vi "S4GUI_001.vi"() -> ()   [LabVIEW 2018] (continued)
            n2909 = call "Write WPROT.vi"("error in (no error)"=w7024, "Opt_Selector.lvclass"=w7023, "Instrument in"=w7042) -> ("error out"=w7021:errorcluster, "Instrument out"=w7022:refnum<class "Instrument.lvclass">)  [unwired: 7 in]
            n2910 = call "Write Instrument.lvclass.vi"("error in (no error)"=w7021, "Instrument.lvclass"=w7022, "S4ACS_GUI in"=w7040) -> ("error out"=w7043:errorcluster, "S4ACS_GUI out"=w7044:refnum<class "S4GUI.lvclass">)  [unwired: 7 in]
            n2911 = call-dynamic "Write ciclos.vi"("error in (no error)"=w7043, "ciclos"=u32 0, "S4ACS_GUI in"=w7044) -> ("error out"=w7017:errorcluster, "S4ACS_GUI out"=w7018:refnum<class "S4GUI.lvclass">)  [unwired: 7 in]
          }
          frame Enabled {
            w7133 = FALSE ("Wait Until Done")
            n2912 = call <vilib>:"Application Directory.vi"() -> ("Application Directory"=w7136:path)
            n2913 = Build Path(base path=w7136, name or relative path="MsgAbortSync.vi") -> (appended path=w7137:path)
            n2914 = Open VI Reference(vi path=w7137, error in (no error)=w7131) -> (vi reference=w7135:refnum<vi>, error out=w7134:errorcluster)  [unwired: 4 in]
            n2915 = invoke class="VI" method="Run VI"(reference=w7135, error in=w7134, "Wait until done"=w7133, "Auto Dispose Ref"=w7133) -> (error out=w7130:errorcluster)  [unwired: 1 in, 4 out]
          }
        }
        n2916 = property on="#Cycles Done" class="Slide (strict)"(error in=w7011, "Scale.Maximum"=w7013, "Scale.Minimum"=w7013) -> (error out=w7014:errorcluster)  [unwired: 1 in, 1 out]
      }
      event "Pause SM": Value Change {
        n2917 = event-data() -> ()  [unwired: 1 in, 6 out]
        n2918 = disable-structure shown="Enabled" {
          disable-tunnel: w7141 -> [w7153 w7162]
          disable-tunnel: w7140 -> [w7152 w7163]
          disable-tunnel: [w7143 w7162] -> w7139
          disable-tunnel: [w7142 w7161] -> w7138
          frame Disabled {
            n2919 = disable-structure shown="Enabled" {
              disable-tunnel: w7153 -> [w7157 w7160]
              disable-tunnel: w7152 -> [w7156 w7159]
              disable-tunnel: [w7155 w7160] -> w7146
              disable-tunnel: [w7154 w7159] -> w7145
              frame Disabled {
                n2920 = call-dynamic "Write paused.vi"("error in (no error)"=w7156, "paused"=TRUE ("stopped"), "S4ACS_GUI in"=w7157) -> ("error out"=w7154:errorcluster, "S4ACS_GUI out"=w7155:refnum<class "S4GUI.lvclass">)  [unwired: 7 in]
              }
              frame Enabled {
              }
            }
            n2921 = call-dynamic "Read Obs_state.vi"("error in (no error)"=w7145, "S4ACS_GUI in"=w7146) -> ("error out"=w7149:errorcluster, "Obs_state"=w7151:u32, "S4ACS_GUI out"=w7150:refnum<class "S4GUI.lvclass">)  [unwired: 7 in]
            n2922 = call-dynamic "Write Obs_prevstate.vi"("error in (no error)"=w7149, "Obs_prevstate"=w7151, "S4ACS_GUI in"=w7150) -> ("error out"=w7147:errorcluster, "S4ACS_GUI out"=w7148:refnum<class "S4GUI.lvclass">)  [unwired: 7 in]
            n2923 = call-dynamic "Write Obs_state.vi"("error in (no error)"=w7147, "Obs_state"=u32 400, "S4ACS_GUI in"=w7148) -> ("error out"=w7142:errorcluster, "S4ACS_GUI out"=w7143:refnum<class "S4GUI.lvclass">)  [unwired: 7 in]
          }
          frame Enabled {
            w7165 = FALSE ("Wait Until Done")
            n2924 = call <vilib>:"Application Directory.vi"() -> ("Application Directory"=w7168:path)
            n2925 = Build Path(base path=w7168, name or relative path="MsgPauseSync.vi") -> (appended path=w7169:path)
            n2926 = Open VI Reference(vi path=w7169, error in (no error)=w7163) -> (vi reference=w7167:refnum<vi>, error out=w7166:errorcluster)  [unwired: 4 in]
            n2927 = invoke class="VI" method="Run VI"(reference=w7167, error in=w7166, "Wait until done"=w7165, "Auto Dispose Ref"=w7165) -> (error out=w7161:errorcluster)  [unwired: 1 in, 4 out]
          }
        }
      }
      event "Abort ch1": Value Change {
        n2928 = event-data() -> ()  [unwired: 1 in, 6 out]
        n2929 = disable-structure shown="Enabled" {
          disable-tunnel: w7173 -> [w7206 w7228]
          disable-tunnel: w7172 -> [w7204 w7221]
          disable-tunnel: [w7186 w7220] -> w7171
          disable-tunnel: [w7174 w7228] -> w7170
          frame Disabled {
            # "Para movimento \nda lamina retardadora"
            # "Restaura a última sequência de lâminas"
            n2930 = call-dynamic "Read AcquisitionA.vi"("error in (no error)"=w7204, "S4ACS_GUI in"=w7206) -> ("error out"=w7209:errorcluster, "Acquisition.lvclass"=w7208:refnum<class "Acquisition.lvclass">, "S4ACS_GUI out"=w7205:refnum<class "S4GUI.lvclass">)  [unwired: 7 in]
            n2931 = call-dynamic "Read Channel.vi"("error in (no error)"=w7209, "Acquisition in"=w7208) -> ("error out"=w7211:errorcluster, "Channel.lvclass"=w7210:refnum<class "Channel.lvclass">, "Acquisition out"=w7217:refnum<class "Acquisition.lvclass">)  [unwired: 7 in]
            n2932 = call-dynamic "Read State Machine.vi"("error in (no error)"=w7211, "Device in"=w7210) -> ("error out"=w7213:errorcluster, "State Machine.lvclass"=w7212:refnum<class "State Machine.lvclass">, "Device out"=w7215:refnum<class "Channel.lvclass">)  [unwired: 7 in]
            n2933 = call "Next State.vi"("error in (no error)"=w7213, "New_State"=u32 80, "State Machine in"=w7212) -> ("error out"=w7216:errorcluster, "State Machine out"=w7214:refnum<class "State Machine.lvclass">)  [unwired: 7 in]
            n2934 = call-dynamic "Write State Machine.vi"("error in (no error)"=w7216, "State Machine.lvclass"=w7214, "Device in"=w7215) -> ("error out"=w7218:errorcluster, "Device out"=w7219:refnum<class "Channel.lvclass">)  [unwired: 7 in]
            n2935 = call-dynamic "Write Channel.vi"("error in (no error)"=w7218, "Channel.lvclass"=w7219, "Acquisition in"=w7217) -> ("error out"=w7201:errorcluster, "Acquisition out"=w7202:refnum<class "Acquisition.lvclass">)  [unwired: 7 in]
            n2936 = call-dynamic "Write Acq_state.vi"("error in (no error)"=w7201, "Acq_state"=u32 0, "Acquisition in"=w7202) -> ("error out"=w7200:errorcluster, "Acquisition out"=w7199:refnum<class "Acquisition.lvclass">)  [unwired: 7 in]
            n2937 = call-dynamic "Write AcquisitionA.vi"("error in (no error)"=w7200, "Acquisition.lvclass"=w7199, "S4ACS_GUI in"=w7205) -> ("error out"=w7187:errorcluster, "S4ACS_GUI out"=w7185:refnum<class "S4GUI.lvclass">)  [unwired: 7 in]
            n2938 = call "Read Instrument.lvclass.vi"("error in (no error)"=w7187, "S4ACS_GUI in"=w7185) -> ("error out"=w7194:errorcluster, "Instrument.lvclass"=w7197:refnum<class "Instrument.lvclass">, "S4ACS_GUI out"=w7198:refnum<class "S4GUI.lvclass">)  [unwired: 7 in]
            n2939 = call "Read WPROT.vi"("error in (no error)"=w7194, "Instrument in"=w7197) -> ("error out"=w7193:errorcluster, "Opt_Selector.lvclass"=w7195:refnum<class "Opt_Selector.lvclass">, "Instrument out"=w7196:refnum<class "Instrument.lvclass">)  [unwired: 7 in]
            n2940 = call-dynamic "Read sequencia_ant.vi"("error in (no error)"=w7193, "Opt_Selector in"=w7195) -> ("error out"=w7189:errorcluster, "sequencia_ant"=w7188:u16, "Opt_Selector out"=w7190:refnum<class "Opt_Selector.lvclass">)  [unwired: 7 in]
            n2941 = call-dynamic "Write sequencia.vi"("error in (no error)"=w7189, "sequencia"=w7188, "Opt_Selector in"=w7190) -> ("error out"=w7178:errorcluster, "Opt_Selector out"=w7179:refnum<class "Opt_Selector.lvclass">)  [unwired: 7 in]
            n2942 = call-dynamic "Read State Machine.vi"("error in (no error)"=w7178, "Device in"=w7179) -> ("error out"=w7181:errorcluster, "State Machine.lvclass"=w7184:refnum<class "State Machine.lvclass">, "Device out"=w7177:refnum<class "Opt_Selector.lvclass">)  [unwired: 7 in]
            n2943 = call "Next State.vi"("error in (no error)"=w7181, "New_State"=10, "State Machine in"=w7184) -> ("error out"=w7180:errorcluster, "State Machine out"=w7183:refnum<class "State Machine.lvclass">)  [unwired: 7 in]
            n2944 = call-dynamic "Write State Machine.vi"("error in (no error)"=w7180, "State Machine.lvclass"=w7183, "Device in"=w7177) -> ("error out"=w7175:errorcluster, "Device out"=w7176:refnum<class "Opt_Selector.lvclass">)  [unwired: 7 in]
            n2945 = call "Write WPROT.vi"("error in (no error)"=w7175, "Opt_Selector.lvclass"=w7176, "Instrument in"=w7196) -> ("error out"=w7192:errorcluster, "Instrument out"=w7191:refnum<class "Instrument.lvclass">)  [unwired: 7 in]
            n2946 = call "Write Instrument.lvclass.vi"("error in (no error)"=w7192, "Instrument.lvclass"=w7191, "S4ACS_GUI in"=w7198) -> ("error out"=w7186:errorcluster, "S4ACS_GUI out"=w7174:refnum<class "S4GUI.lvclass">)  [unwired: 7 in]
          }
          frame Enabled {
            w7223 = FALSE ("Wait Until Done")
            n2947 = call <vilib>:"Application Directory.vi"() -> ("Application Directory"=w7226:path)
            n2948 = Build Path(base path=w7226, name or relative path="MsgAbort1.vi") -> (appended path=w7227:path)
            n2949 = Open VI Reference(vi path=w7227, error in (no error)=w7221) -> (vi reference=w7225:refnum<vi>, error out=w7224:errorcluster)  [unwired: 4 in]
            n2950 = invoke class="VI" method="Run VI"(reference=w7225, error in=w7224, "Wait until done"=w7223, "Auto Dispose Ref"=w7223) -> (error out=w7220:errorcluster)  [unwired: 1 in, 4 out]
          }
        }
      }
      event "Abort ch2": Value Change {
        n2951 = event-data() -> ()  [unwired: 1 in, 6 out]
        n2952 = disable-structure shown="Enabled" {
          disable-tunnel: w7232 -> [w7265 w7280]
          disable-tunnel: w7231 -> [w7263 w7281]
          disable-tunnel: [w7245 w7279] -> w7230
          disable-tunnel: [w7233 w7280] -> w7229
          frame Disabled {
            # "Para movimento \nda lamina retardadora"
            # "Restaura a última sequência de lâminas"
            n2953 = call "Read AcquisitionB.vi"("error in (no error)"=w7263, "S4ACS_GUI in"=w7265) -> ("error out"=w7268:errorcluster, "Acquisition.lvclass"=w7267:refnum<class "Acquisition.lvclass">, "S4ACS_GUI out"=w7264:refnum<class "S4GUI.lvclass">)  [unwired: 7 in]
            n2954 = call-dynamic "Read Channel.vi"("error in (no error)"=w7268, "Acquisition in"=w7267) -> ("error out"=w7270:errorcluster, "Channel.lvclass"=w7269:refnum<class "Channel.lvclass">, "Acquisition out"=w7276:refnum<class "Acquisition.lvclass">)  [unwired: 7 in]
            n2955 = call-dynamic "Read State Machine.vi"("error in (no error)"=w7270, "Device in"=w7269) -> ("error out"=w7272:errorcluster, "State Machine.lvclass"=w7271:refnum<class "State Machine.lvclass">, "Device out"=w7274:refnum<class "Channel.lvclass">)  [unwired: 7 in]
            n2956 = call "Next State.vi"("error in (no error)"=w7272, "New_State"=u32 80, "State Machine in"=w7271) -> ("error out"=w7275:errorcluster, "State Machine out"=w7273:refnum<class "State Machine.lvclass">)  [unwired: 7 in]
            n2957 = call-dynamic "Write State Machine.vi"("error in (no error)"=w7275, "State Machine.lvclass"=w7273, "Device in"=w7274) -> ("error out"=w7277:errorcluster, "Device out"=w7278:refnum<class "Channel.lvclass">)  [unwired: 7 in]
            n2958 = call-dynamic "Write Channel.vi"("error in (no error)"=w7277, "Channel.lvclass"=w7278, "Acquisition in"=w7276) -> ("error out"=w7260:errorcluster, "Acquisition out"=w7261:refnum<class "Acquisition.lvclass">)  [unwired: 7 in]
            n2959 = call-dynamic "Write Acq_state.vi"("error in (no error)"=w7260, "Acq_state"=u32 0, "Acquisition in"=w7261) -> ("error out"=w7259:errorcluster, "Acquisition out"=w7258:refnum<class "Acquisition.lvclass">)  [unwired: 7 in]
            n2960 = call "Write AcquisitionB.vi"("error in (no error)"=w7259, "Acquisition.lvclass"=w7258, "S4ACS_GUI in"=w7264) -> ("error out"=w7246:errorcluster, "S4ACS_GUI out"=w7244:refnum<class "S4GUI.lvclass">)  [unwired: 7 in]
            n2961 = call "Read Instrument.lvclass.vi"("error in (no error)"=w7246, "S4ACS_GUI in"=w7244) -> ("error out"=w7253:errorcluster, "Instrument.lvclass"=w7256:refnum<class "Instrument.lvclass">, "S4ACS_GUI out"=w7257:refnum<class "S4GUI.lvclass">)  [unwired: 7 in]
            n2962 = call "Read WPROT.vi"("error in (no error)"=w7253, "Instrument in"=w7256) -> ("error out"=w7252:errorcluster, "Opt_Selector.lvclass"=w7254:refnum<class "Opt_Selector.lvclass">, "Instrument out"=w7255:refnum<class "Instrument.lvclass">)  [unwired: 7 in]
            n2963 = call-dynamic "Read sequencia_ant.vi"("error in (no error)"=w7252, "Opt_Selector in"=w7254) -> ("error out"=w7248:errorcluster, "sequencia_ant"=w7247:u16, "Opt_Selector out"=w7249:refnum<class "Opt_Selector.lvclass">)  [unwired: 7 in]
            n2964 = call-dynamic "Write sequencia.vi"("error in (no error)"=w7248, "sequencia"=w7247, "Opt_Selector in"=w7249) -> ("error out"=w7237:errorcluster, "Opt_Selector out"=w7238:refnum<class "Opt_Selector.lvclass">)  [unwired: 7 in]
            n2965 = call-dynamic "Read State Machine.vi"("error in (no error)"=w7237, "Device in"=w7238) -> ("error out"=w7240:errorcluster, "State Machine.lvclass"=w7243:refnum<class "State Machine.lvclass">, "Device out"=w7236:refnum<class "Opt_Selector.lvclass">)  [unwired: 7 in]
            n2966 = call "Next State.vi"("error in (no error)"=w7240, "New_State"=10, "State Machine in"=w7243) -> ("error out"=w7239:errorcluster, "State Machine out"=w7242:refnum<class "State Machine.lvclass">)  [unwired: 7 in]
            n2967 = call-dynamic "Write State Machine.vi"("error in (no error)"=w7239, "State Machine.lvclass"=w7242, "Device in"=w7236) -> ("error out"=w7234:errorcluster, "Device out"=w7235:refnum<class "Opt_Selector.lvclass">)  [unwired: 7 in]
            n2968 = call "Write WPROT.vi"("error in (no error)"=w7234, "Opt_Selector.lvclass"=w7235, "Instrument in"=w7255) -> ("error out"=w7251:errorcluster, "Instrument out"=w7250:refnum<class "Instrument.lvclass">)  [unwired: 7 in]
            n2969 = call "Write Instrument.lvclass.vi"("error in (no error)"=w7251, "Instrument.lvclass"=w7250, "S4ACS_GUI in"=w7257) -> ("error out"=w7245:errorcluster, "S4ACS_GUI out"=w7233:refnum<class "S4GUI.lvclass">)  [unwired: 7 in]
          }
          frame Enabled {
            w7283 = FALSE ("Wait Until Done")
            n2970 = call <vilib>:"Application Directory.vi"() -> ("Application Directory"=w7286:path)
            n2971 = Build Path(base path=w7286, name or relative path="MsgAbort2.vi") -> (appended path=w7287:path)
            n2972 = Open VI Reference(vi path=w7287, error in (no error)=w7281) -> (vi reference=w7285:refnum<vi>, error out=w7284:errorcluster)  [unwired: 4 in]
            n2973 = invoke class="VI" method="Run VI"(reference=w7285, error in=w7284, "Wait until done"=w7283, "Auto Dispose Ref"=w7283) -> (error out=w7279:errorcluster)  [unwired: 1 in, 4 out]
          }
        }
      }
      event "Abort ch3": Value Change {
        n2974 = event-data() -> ()  [unwired: 1 in, 6 out]
        n2975 = disable-structure shown="Enabled" {
          disable-tunnel: w7291 -> [w7324 w7339]
          disable-tunnel: w7290 -> [w7322 w7340]
          disable-tunnel: [w7304 w7338] -> w7289
          disable-tunnel: [w7292 w7339] -> w7288
          frame Disabled {
            # "Para movimento \nda lamina retardadora"
            # "Restaura a última sequência de lâminas"
            n2976 = call-dynamic "Read AcquisitionC.vi"("error in (no error)"=w7322, "S4ACS_GUI in"=w7324) -> ("error out"=w7327:errorcluster, "Acquisition.lvclass"=w7326:refnum<class "Acquisition.lvclass">, "S4ACS_GUI out"=w7323:refnum<class "S4GUI.lvclass">)  [unwired: 7 in]
            n2977 = call-dynamic "Read Channel.vi"("error in (no error)"=w7327, "Acquisition in"=w7326) -> ("error out"=w7329:errorcluster, "Channel.lvclass"=w7328:refnum<class "Channel.lvclass">, "Acquisition out"=w7335:refnum<class "Acquisition.lvclass">)  [unwired: 7 in]
            n2978 = call-dynamic "Read State Machine.vi"("error in (no error)"=w7329, "Device in"=w7328) -> ("error out"=w7331:errorcluster, "State Machine.lvclass"=w7330:refnum<class "State Machine.lvclass">, "Device out"=w7333:refnum<class "Channel.lvclass">)  [unwired: 7 in]
            n2979 = call "Next State.vi"("error in (no error)"=w7331, "New_State"=u32 80, "State Machine in"=w7330) -> ("error out"=w7334:errorcluster, "State Machine out"=w7332:refnum<class "State Machine.lvclass">)  [unwired: 7 in]
            n2980 = call-dynamic "Write State Machine.vi"("error in (no error)"=w7334, "State Machine.lvclass"=w7332, "Device in"=w7333) -> ("error out"=w7336:errorcluster, "Device out"=w7337:refnum<class "Channel.lvclass">)  [unwired: 7 in]
            n2981 = call-dynamic "Write Channel.vi"("error in (no error)"=w7336, "Channel.lvclass"=w7337, "Acquisition in"=w7335) -> ("error out"=w7319:errorcluster, "Acquisition out"=w7320:refnum<class "Acquisition.lvclass">)  [unwired: 7 in]
            n2982 = call-dynamic "Write Acq_state.vi"("error in (no error)"=w7319, "Acq_state"=u32 0, "Acquisition in"=w7320) -> ("error out"=w7318:errorcluster, "Acquisition out"=w7317:refnum<class "Acquisition.lvclass">)  [unwired: 7 in]
            n2983 = call-dynamic "Write AcquisitionC.vi"("error in (no error)"=w7318, "Acquisition.lvclass"=w7317, "S4ACS_GUI in"=w7323) -> ("error out"=w7305:errorcluster, "S4ACS_GUI out"=w7303:refnum<class "S4GUI.lvclass">)  [unwired: 7 in]
            n2984 = call "Read Instrument.lvclass.vi"("error in (no error)"=w7305, "S4ACS_GUI in"=w7303) -> ("error out"=w7312:errorcluster, "Instrument.lvclass"=w7315:refnum<class "Instrument.lvclass">, "S4ACS_GUI out"=w7316:refnum<class "S4GUI.lvclass">)  [unwired: 7 in]
            n2985 = call "Read WPROT.vi"("error in (no error)"=w7312, "Instrument in"=w7315) -> ("error out"=w7311:errorcluster, "Opt_Selector.lvclass"=w7313:refnum<class "Opt_Selector.lvclass">, "Instrument out"=w7314:refnum<class "Instrument.lvclass">)  [unwired: 7 in]
            n2986 = call-dynamic "Read sequencia_ant.vi"("error in (no error)"=w7311, "Opt_Selector in"=w7313) -> ("error out"=w7307:errorcluster, "sequencia_ant"=w7306:u16, "Opt_Selector out"=w7308:refnum<class "Opt_Selector.lvclass">)  [unwired: 7 in]
            n2987 = call-dynamic "Write sequencia.vi"("error in (no error)"=w7307, "sequencia"=w7306, "Opt_Selector in"=w7308) -> ("error out"=w7296:errorcluster, "Opt_Selector out"=w7297:refnum<class "Opt_Selector.lvclass">)  [unwired: 7 in]
            n2988 = call-dynamic "Read State Machine.vi"("error in (no error)"=w7296, "Device in"=w7297) -> ("error out"=w7299:errorcluster, "State Machine.lvclass"=w7302:refnum<class "State Machine.lvclass">, "Device out"=w7295:refnum<class "Opt_Selector.lvclass">)  [unwired: 7 in]
            n2989 = call "Next State.vi"("error in (no error)"=w7299, "New_State"=10, "State Machine in"=w7302) -> ("error out"=w7298:errorcluster, "State Machine out"=w7301:refnum<class "State Machine.lvclass">)  [unwired: 7 in]
            n2990 = call-dynamic "Write State Machine.vi"("error in (no error)"=w7298, "State Machine.lvclass"=w7301, "Device in"=w7295) -> ("error out"=w7293:errorcluster, "Device out"=w7294:refnum<class "Opt_Selector.lvclass">)  [unwired: 7 in]
            n2991 = call "Write WPROT.vi"("error in (no error)"=w7293, "Opt_Selector.lvclass"=w7294, "Instrument in"=w7314) -> ("error out"=w7310:errorcluster, "Instrument out"=w7309:refnum<class "Instrument.lvclass">)  [unwired: 7 in]
            n2992 = call "Write Instrument.lvclass.vi"("error in (no error)"=w7310, "Instrument.lvclass"=w7309, "S4ACS_GUI in"=w7316) -> ("error out"=w7304:errorcluster, "S4ACS_GUI out"=w7292:refnum<class "S4GUI.lvclass">)  [unwired: 7 in]
          }
          frame Enabled {
            w7342 = FALSE ("Wait Until Done")
            n2993 = call <vilib>:"Application Directory.vi"() -> ("Application Directory"=w7345:path)
            n2994 = Build Path(base path=w7345, name or relative path="MsgAbort3.vi") -> (appended path=w7346:path)
            n2995 = Open VI Reference(vi path=w7346, error in (no error)=w7340) -> (vi reference=w7344:refnum<vi>, error out=w7343:errorcluster)  [unwired: 4 in]
            n2996 = invoke class="VI" method="Run VI"(reference=w7344, error in=w7343, "Wait until done"=w7342, "Auto Dispose Ref"=w7342) -> (error out=w7338:errorcluster)  [unwired: 1 in, 4 out]
          }
        }
      }
      event "Abort ch4": Value Change {
        n2997 = event-data() -> ()  [unwired: 1 in, 6 out]
        n2998 = disable-structure shown="Enabled" {
          disable-tunnel: w7350 -> [w7383 w7398]
          disable-tunnel: w7349 -> [w7381 w7399]
          disable-tunnel: [w7363 w7397] -> w7348
          disable-tunnel: [w7351 w7398] -> w7347
          frame Disabled {
            # "Para movimento \nda lamina retardadora"
            # "Restaura a última sequência de lâminas"
            n2999 = call-dynamic "Read AcquisitionD.vi"("error in (no error)"=w7381, "S4ACS_GUI in"=w7383) -> ("error out"=w7386:errorcluster, "Acquisition.lvclass"=w7385:refnum<class "Acquisition.lvclass">, "S4ACS_GUI out"=w7382:refnum<class "S4GUI.lvclass">)  [unwired: 7 in]
            n3000 = call-dynamic "Read Channel.vi"("error in (no error)"=w7386, "Acquisition in"=w7385) -> ("error out"=w7388:errorcluster, "Channel.lvclass"=w7387:refnum<class "Channel.lvclass">, "Acquisition out"=w7394:refnum<class "Acquisition.lvclass">)  [unwired: 7 in]
            n3001 = call-dynamic "Read State Machine.vi"("error in (no error)"=w7388, "Device in"=w7387) -> ("error out"=w7390:errorcluster, "State Machine.lvclass"=w7389:refnum<class "State Machine.lvclass">, "Device out"=w7392:refnum<class "Channel.lvclass">)  [unwired: 7 in]
            n3002 = call "Next State.vi"("error in (no error)"=w7390, "New_State"=u32 80, "State Machine in"=w7389) -> ("error out"=w7393:errorcluster, "State Machine out"=w7391:refnum<class "State Machine.lvclass">)  [unwired: 7 in]
            n3003 = call-dynamic "Write State Machine.vi"("error in (no error)"=w7393, "State Machine.lvclass"=w7391, "Device in"=w7392) -> ("error out"=w7395:errorcluster, "Device out"=w7396:refnum<class "Channel.lvclass">)  [unwired: 7 in]
            n3004 = call-dynamic "Write Channel.vi"("error in (no error)"=w7395, "Channel.lvclass"=w7396, "Acquisition in"=w7394) -> ("error out"=w7378:errorcluster, "Acquisition out"=w7379:refnum<class "Acquisition.lvclass">)  [unwired: 7 in]
            n3005 = call-dynamic "Write Acq_state.vi"("error in (no error)"=w7378, "Acq_state"=u32 0, "Acquisition in"=w7379) -> ("error out"=w7377:errorcluster, "Acquisition out"=w7376:refnum<class "Acquisition.lvclass">)  [unwired: 7 in]
            n3006 = call-dynamic "Write AcquisitionD.vi"("error in (no error)"=w7377, "Acquisition.lvclass"=w7376, "S4ACS_GUI in"=w7382) -> ("error out"=w7364:errorcluster, "S4ACS_GUI out"=w7362:refnum<class "S4GUI.lvclass">)  [unwired: 7 in]
            n3007 = call "Read Instrument.lvclass.vi"("error in (no error)"=w7364, "S4ACS_GUI in"=w7362) -> ("error out"=w7371:errorcluster, "Instrument.lvclass"=w7374:refnum<class "Instrument.lvclass">, "S4ACS_GUI out"=w7375:refnum<class "S4GUI.lvclass">)  [unwired: 7 in]
            n3008 = call "Read WPROT.vi"("error in (no error)"=w7371, "Instrument in"=w7374) -> ("error out"=w7370:errorcluster, "Opt_Selector.lvclass"=w7372:refnum<class "Opt_Selector.lvclass">, "Instrument out"=w7373:refnum<class "Instrument.lvclass">)  [unwired: 7 in]
            n3009 = call-dynamic "Read sequencia_ant.vi"("error in (no error)"=w7370, "Opt_Selector in"=w7372) -> ("error out"=w7366:errorcluster, "sequencia_ant"=w7365:u16, "Opt_Selector out"=w7367:refnum<class "Opt_Selector.lvclass">)  [unwired: 7 in]
            n3010 = call-dynamic "Write sequencia.vi"("error in (no error)"=w7366, "sequencia"=w7365, "Opt_Selector in"=w7367) -> ("error out"=w7355:errorcluster, "Opt_Selector out"=w7356:refnum<class "Opt_Selector.lvclass">)  [unwired: 7 in]
            n3011 = call-dynamic "Read State Machine.vi"("error in (no error)"=w7355, "Device in"=w7356) -> ("error out"=w7358:errorcluster, "State Machine.lvclass"=w7361:refnum<class "State Machine.lvclass">, "Device out"=w7354:refnum<class "Opt_Selector.lvclass">)  [unwired: 7 in]
            n3012 = call "Next State.vi"("error in (no error)"=w7358, "New_State"=10, "State Machine in"=w7361) -> ("error out"=w7357:errorcluster, "State Machine out"=w7360:refnum<class "State Machine.lvclass">)  [unwired: 7 in]
            n3013 = call-dynamic "Write State Machine.vi"("error in (no error)"=w7357, "State Machine.lvclass"=w7360, "Device in"=w7354) -> ("error out"=w7352:errorcluster, "Device out"=w7353:refnum<class "Opt_Selector.lvclass">)  [unwired: 7 in]
            n3014 = call "Write WPROT.vi"("error in (no error)"=w7352, "Opt_Selector.lvclass"=w7353, "Instrument in"=w7373) -> ("error out"=w7369:errorcluster, "Instrument out"=w7368:refnum<class "Instrument.lvclass">)  [unwired: 7 in]
            n3015 = call "Write Instrument.lvclass.vi"("error in (no error)"=w7369, "Instrument.lvclass"=w7368, "S4ACS_GUI in"=w7375) -> ("error out"=w7363:errorcluster, "S4ACS_GUI out"=w7351:refnum<class "S4GUI.lvclass">)  [unwired: 7 in]
          }
          frame Enabled {
            w7401 = FALSE ("Wait Until Done")
            n3016 = call <vilib>:"Application Directory.vi"() -> ("Application Directory"=w7404:path)
            n3017 = Build Path(base path=w7404, name or relative path="MsgAbort4.vi") -> (appended path=w7405:path)
            n3018 = Open VI Reference(vi path=w7405, error in (no error)=w7399) -> (vi reference=w7403:refnum<vi>, error out=w7402:errorcluster)  [unwired: 4 in]
            n3019 = invoke class="VI" method="Run VI"(reference=w7403, error in=w7402, "Wait until done"=w7401, "Auto Dispose Ref"=w7401) -> (error out=w7397:errorcluster)  [unwired: 1 in, 4 out]
          }
        }
      }
      event "SyncBox": Value Change {
        n3020 = event-data() -> ()  [unwired: 1 in, 4 out]
        n3021 = call-dynamic "Read Sync Box.lvclass.vi"("error in (no error)"=w7408, "SPARC4_AC in"=w7409) -> ("error out"=w7424:errorcluster, "Sync Box.lvclass"=w7425:refnum<class "Sync Box.lvclass">, "SPARC4_AC out"=w7413:refnum<class "S4GUI.lvclass">)  [unwired: 7 in]
        n3022 = call-dynamic "Read Trigger.lvclass.vi"("error in (no error)"=w7424, "Sync Box in"=w7425) -> ("error out"=w7422:errorcluster, "Trigger.lvclass"=w7423:refnum<class "Trigger.lvclass">, "Sync Box out"=w7416:refnum<class "Sync Box.lvclass">)  [unwired: 7 in]
        n3023 = call-dynamic "Read State Machine.vi"("error in (no error)"=w7422, "Device in"=w7423) -> ("error out"=w7420:errorcluster, "State Machine.lvclass"=w7421:refnum<class "State Machine.lvclass">, "Device out"=w7417:refnum<class "Trigger.lvclass">)  [unwired: 7 in]
        n3024 = call "Next State.vi"("error in (no error)"=w7420, "New_State"=u32 1, "State Machine in"=w7421) -> ("error out"=w7415:errorcluster, "State Machine out"=w7418:refnum<class "State Machine.lvclass">)  [unwired: 7 in]
        n3025 = call-dynamic "Write State Machine.vi"("error in (no error)"=w7415, "State Machine.lvclass"=w7418, "Device in"=w7417) -> ("error out"=w7411:errorcluster, "Device out"=w7410:refnum<class "Trigger.lvclass">)  [unwired: 7 in]
        n3026 = call-dynamic "Write Trigger.lvclass.vi"("error in (no error)"=w7411, "Trigger.lvclass"=w7410, "Sync Box in"=w7416) -> ("error out"=w7412:errorcluster, "Sync Box out"=w7414:refnum<class "Sync Box.lvclass">)  [unwired: 7 in]
        n3027 = call-dynamic "Write Sync Box.lvclass.vi"("error in (no error)"=w7412, "Sync Box.lvclass"=w7414, "SPARC4_AC in"=w7413) -> ("error out"=w7407:errorcluster, "SPARC4_AC out"=w7406:refnum<class "S4GUI.lvclass">)  [unwired: 7 in]
      }
      event "Fire manual", "Fire": Value Change {
        n3028 = event-data() -> ()  [unwired: 1 in, 4 out]
        n3029 = call-dynamic "Read Sync Box.lvclass.vi"("error in (no error)"=w7428, "SPARC4_AC in"=w7429) -> ("error out"=w7444:errorcluster, "Sync Box.lvclass"=w7445:refnum<class "Sync Box.lvclass">, "SPARC4_AC out"=w7433:refnum<class "S4GUI.lvclass">)  [unwired: 7 in]
        n3030 = call-dynamic "Read Trigger.lvclass.vi"("error in (no error)"=w7444, "Sync Box in"=w7445) -> ("error out"=w7442:errorcluster, "Trigger.lvclass"=w7443:refnum<class "Trigger.lvclass">, "Sync Box out"=w7436:refnum<class "Sync Box.lvclass">)  [unwired: 7 in]
        n3031 = call-dynamic "Read State Machine.vi"("error in (no error)"=w7442, "Device in"=w7443) -> ("error out"=w7440:errorcluster, "State Machine.lvclass"=w7441:refnum<class "State Machine.lvclass">, "Device out"=w7437:refnum<class "Trigger.lvclass">)  [unwired: 7 in]
        n3032 = call "Next State.vi"("error in (no error)"=w7440, "New_State"=u32 40, "State Machine in"=w7441) -> ("error out"=w7435:errorcluster, "State Machine out"=w7438:refnum<class "State Machine.lvclass">)  [unwired: 7 in]
        n3033 = call-dynamic "Write State Machine.vi"("error in (no error)"=w7435, "State Machine.lvclass"=w7438, "Device in"=w7437) -> ("error out"=w7431:errorcluster, "Device out"=w7430:refnum<class "Trigger.lvclass">)  [unwired: 7 in]
        n3034 = call-dynamic "Write Trigger.lvclass.vi"("error in (no error)"=w7431, "Trigger.lvclass"=w7430, "Sync Box in"=w7436) -> ("error out"=w7432:errorcluster, "Sync Box out"=w7434:refnum<class "Sync Box.lvclass">)  [unwired: 7 in]
        n3035 = call-dynamic "Write Sync Box.lvclass.vi"("error in (no error)"=w7432, "Sync Box.lvclass"=w7434, "SPARC4_AC in"=w7433) -> ("error out"=w7427:errorcluster, "SPARC4_AC out"=w7426:refnum<class "S4GUI.lvclass">)  [unwired: 7 in]
      }
      event "Select Trigger Mode": Value Change {
        n3036 = event-data() -> ("NewVal"=w7447:bool)  [unwired: 1 in, 2 out]
        n3037 = call-dynamic "Read Sync Box.lvclass.vi"("error in (no error)"=w7455, "SPARC4_AC in"=w7456) -> ("error out"=w7467:errorcluster, "Sync Box.lvclass"=w7468:refnum<class "Sync Box.lvclass">, "SPARC4_AC out"=w7460:refnum<class "S4GUI.lvclass">)  [unwired: 7 in]
        n3038 = call-dynamic "Read Trigger.lvclass.vi"("error in (no error)"=w7467, "Sync Box in"=w7468) -> ("error out"=w7448:errorcluster, "Trigger.lvclass"=w7451:refnum<class "Trigger.lvclass">, "Sync Box out"=w7463:refnum<class "Sync Box.lvclass">)  [unwired: 7 in]
        n3039 = call-dynamic "Write Trigger Mode Target.vi"("error in (no error)"=w7448, "Trigger Mode Target"=w7447, "Trigger in"=w7451) -> ("error out"=w7449:errorcluster, "Trigger out"=w7450:refnum<class "Trigger.lvclass">)  [unwired: 7 in]
        n3040 = call-dynamic "Read State Machine.vi"("error in (no error)"=w7449, "Device in"=w7450) -> ("error out"=w7452:errorcluster, "State Machine.lvclass"=w7453:refnum<class "State Machine.lvclass">, "Device out"=w7464:refnum<class "Trigger.lvclass">)  [unwired: 7 in]
        n3041 = call "Next State.vi"("error in (no error)"=w7452, "New_State"=u32 30, "State Machine in"=w7453) -> ("error out"=w7462:errorcluster, "State Machine out"=w7465:refnum<class "State Machine.lvclass">)  [unwired: 7 in]
        n3042 = call-dynamic "Write State Machine.vi"("error in (no error)"=w7462, "State Machine.lvclass"=w7465, "Device in"=w7464) -> ("error out"=w7458:errorcluster, "Device out"=w7457:refnum<class "Trigger.lvclass">)  [unwired: 7 in]
        n3043 = call-dynamic "Write Trigger.lvclass.vi"("error in (no error)"=w7458, "Trigger.lvclass"=w7457, "Sync Box in"=w7463) -> ("error out"=w7459:errorcluster, "Sync Box out"=w7461:refnum<class "Sync Box.lvclass">)  [unwired: 7 in]
        n3044 = call-dynamic "Write Sync Box.lvclass.vi"("error in (no error)"=w7459, "Sync Box.lvclass"=w7461, "SPARC4_AC in"=w7460) -> ("error out"=w7454:errorcluster, "SPARC4_AC out"=w7446:refnum<class "S4GUI.lvclass">)  [unwired: 7 in]
      }
      event "Set SyncBox": Value Change {
        n3045 = event-data() -> ()  [unwired: 1 in, 4 out]
        n3046 = call-dynamic "Read Sync Box.lvclass.vi"("error in (no error)"=w7471, "SPARC4_AC in"=w7472) -> ("error out"=w7487:errorcluster, "Sync Box.lvclass"=w7488:refnum<class "Sync Box.lvclass">, "SPARC4_AC out"=w7476:refnum<class "S4GUI.lvclass">)  [unwired: 7 in]
        n3047 = call-dynamic "Read Trigger.lvclass.vi"("error in (no error)"=w7487, "Sync Box in"=w7488) -> ("error out"=w7485:errorcluster, "Trigger.lvclass"=w7486:refnum<class "Trigger.lvclass">, "Sync Box out"=w7479:refnum<class "Sync Box.lvclass">)  [unwired: 7 in]
        n3048 = call-dynamic "Read State Machine.vi"("error in (no error)"=w7485, "Device in"=w7486) -> ("error out"=w7483:errorcluster, "State Machine.lvclass"=w7484:refnum<class "State Machine.lvclass">, "Device out"=w7480:refnum<class "Trigger.lvclass">)  [unwired: 7 in]
        n3049 = call "Next State.vi"("error in (no error)"=w7483, "New_State"=u32 10, "State Machine in"=w7484) -> ("error out"=w7478:errorcluster, "State Machine out"=w7481:refnum<class "State Machine.lvclass">)  [unwired: 7 in]
        n3050 = call-dynamic "Write State Machine.vi"("error in (no error)"=w7478, "State Machine.lvclass"=w7481, "Device in"=w7480) -> ("error out"=w7474:errorcluster, "Device out"=w7473:refnum<class "Trigger.lvclass">)  [unwired: 7 in]
        n3051 = call-dynamic "Write Trigger.lvclass.vi"("error in (no error)"=w7474, "Trigger.lvclass"=w7473, "Sync Box in"=w7479) -> ("error out"=w7475:errorcluster, "Sync Box out"=w7477:refnum<class "Sync Box.lvclass">)  [unwired: 7 in]
        n3052 = call-dynamic "Write Sync Box.lvclass.vi"("error in (no error)"=w7475, "Sync Box.lvclass"=w7477, "SPARC4_AC in"=w7476) -> ("error out"=w7470:errorcluster, "SPARC4_AC out"=w7469:refnum<class "S4GUI.lvclass">)  [unwired: 7 in]
      }
      event "Cooler 1": Value Change {
        n3053 = event-data() -> ("NewVal"=w7489:bool)  [unwired: 1 in]
        n3054 = case shown="True" w7489 {
          tunnel: w7493 -> [w7495 w7499]
          tunnel: w7492 -> [w7494 w7498]
          tunnel: [w7494 w7497] -> w7491
          tunnel: [w7495 w7496] -> w7490
          frame False {
          }
          frame True {
            n3055 = call-dynamic "Read AcquisitionA.vi"("error in (no error)"=w7498, "S4ACS_GUI in"=w7499) -> ("error out"=w7514:errorcluster, "Acquisition.lvclass"=w7515:refnum<class "Acquisition.lvclass">, "S4ACS_GUI out"=w7503:refnum<class "S4GUI.lvclass">)  [unwired: 7 in]
            n3056 = call-dynamic "Read Channel.vi"("error in (no error)"=w7514, "Acquisition in"=w7515) -> ("error out"=w7512:errorcluster, "Channel.lvclass"=w7513:refnum<class "Channel.lvclass">, "Acquisition out"=w7506:refnum<class "Acquisition.lvclass">)  [unwired: 7 in]
            n3057 = call-dynamic "Read State Machine.vi"("error in (no error)"=w7512, "Device in"=w7513) -> ("error out"=w7510:errorcluster, "State Machine.lvclass"=w7511:refnum<class "State Machine.lvclass">, "Device out"=w7507:refnum<class "Channel.lvclass">)  [unwired: 7 in]
            n3058 = call "Next State.vi"("error in (no error)"=w7510, "New_State"=u32 30, "State Machine in"=w7511) -> ("error out"=w7505:errorcluster, "State Machine out"=w7508:refnum<class "State Machine.lvclass">)  [unwired: 7 in]
            n3059 = call-dynamic "Write State Machine.vi"("error in (no error)"=w7505, "State Machine.lvclass"=w7508, "Device in"=w7507) -> ("error out"=w7501:errorcluster, "Device out"=w7500:refnum<class "Channel.lvclass">)  [unwired: 7 in]
            n3060 = call-dynamic "Write Channel.vi"("error in (no error)"=w7501, "Channel.lvclass"=w7500, "Acquisition in"=w7506) -> ("error out"=w7502:errorcluster, "Acquisition out"=w7504:refnum<class "Acquisition.lvclass">)  [unwired: 7 in]
            n3061 = call-dynamic "Write AcquisitionA.vi"("error in (no error)"=w7502, "Acquisition.lvclass"=w7504, "S4ACS_GUI in"=w7503) -> ("error out"=w7497:errorcluster, "S4ACS_GUI out"=w7496:refnum<class "S4GUI.lvclass">)  [unwired: 7 in]
          }
        }
      }
      event "Cooler 2": Value Change {
        n3062 = event-data() -> ("NewVal"=w7516:bool)  [unwired: 1 in]
        n3063 = case shown="True" w7516 {
          tunnel: w7520 -> [w7522 w7526]
          tunnel: w7519 -> [w7521 w7525]
          tunnel: [w7521 w7524] -> w7518
          tunnel: [w7522 w7523] -> w7517
          frame False {
          }
          frame True {
            n3064 = call "Read AcquisitionB.vi"("error in (no error)"=w7525, "S4ACS_GUI in"=w7526) -> ("error out"=w7541:errorcluster, "Acquisition.lvclass"=w7542:refnum<class "Acquisition.lvclass">, "S4ACS_GUI out"=w7530:refnum<class "S4GUI.lvclass">)  [unwired: 7 in]
            n3065 = call-dynamic "Read Channel.vi"("error in (no error)"=w7541, "Acquisition in"=w7542) -> ("error out"=w7539:errorcluster, "Channel.lvclass"=w7540:refnum<class "Channel.lvclass">, "Acquisition out"=w7533:refnum<class "Acquisition.lvclass">)  [unwired: 7 in]
            n3066 = call-dynamic "Read State Machine.vi"("error in (no error)"=w7539, "Device in"=w7540) -> ("error out"=w7537:errorcluster, "State Machine.lvclass"=w7538:refnum<class "State Machine.lvclass">, "Device out"=w7534:refnum<class "Channel.lvclass">)  [unwired: 7 in]
            n3067 = call "Next State.vi"("error in (no error)"=w7537, "New_State"=u32 30, "State Machine in"=w7538) -> ("error out"=w7532:errorcluster, "State Machine out"=w7535:refnum<class "State Machine.lvclass">)  [unwired: 7 in]
            n3068 = call-dynamic "Write State Machine.vi"("error in (no error)"=w7532, "State Machine.lvclass"=w7535, "Device in"=w7534) -> ("error out"=w7528:errorcluster, "Device out"=w7527:refnum<class "Channel.lvclass">)  [unwired: 7 in]
            n3069 = call-dynamic "Write Channel.vi"("error in (no error)"=w7528, "Channel.lvclass"=w7527, "Acquisition in"=w7533) -> ("error out"=w7529:errorcluster, "Acquisition out"=w7531:refnum<class "Acquisition.lvclass">)  [unwired: 7 in]
            n3070 = call "Write AcquisitionB.vi"("error in (no error)"=w7529, "Acquisition.lvclass"=w7531, "S4ACS_GUI in"=w7530) -> ("error out"=w7524:errorcluster, "S4ACS_GUI out"=w7523:refnum<class "S4GUI.lvclass">)  [unwired: 7 in]
          }
        }
      }
      event "Cooler 3": Value Change {
        n3071 = event-data() -> ("NewVal"=w7543:bool)  [unwired: 1 in]
        n3072 = case shown="True" w7543 {
          tunnel: w7547 -> [w7549 w7553]
          tunnel: w7546 -> [w7548 w7552]
          tunnel: [w7548 w7551] -> w7545
          tunnel: [w7549 w7550] -> w7544
          frame False {
          }
          frame True {
            n3073 = call-dynamic "Read AcquisitionC.vi"("error in (no error)"=w7552, "S4ACS_GUI in"=w7553) -> ("error out"=w7568:errorcluster, "Acquisition.lvclass"=w7569:refnum<class "Acquisition.lvclass">, "S4ACS_GUI out"=w7557:refnum<class "S4GUI.lvclass">)  [unwired: 7 in]
            n3074 = call-dynamic "Read Channel.vi"("error in (no error)"=w7568, "Acquisition in"=w7569) -> ("error out"=w7566:errorcluster, "Channel.lvclass"=w7567:refnum<class "Channel.lvclass">, "Acquisition out"=w7560:refnum<class "Acquisition.lvclass">)  [unwired: 7 in]
            n3075 = call-dynamic "Read State Machine.vi"("error in (no error)"=w7566, "Device in"=w7567) -> ("error out"=w7564:errorcluster, "State Machine.lvclass"=w7565:refnum<class "State Machine.lvclass">, "Device out"=w7561:refnum<class "Channel.lvclass">)  [unwired: 7 in]
            n3076 = call "Next State.vi"("error in (no error)"=w7564, "New_State"=u32 30, "State Machine in"=w7565) -> ("error out"=w7559:errorcluster, "State Machine out"=w7562:refnum<class "State Machine.lvclass">)  [unwired: 7 in]
            n3077 = call-dynamic "Write State Machine.vi"("error in (no error)"=w7559, "State Machine.lvclass"=w7562, "Device in"=w7561) -> ("error out"=w7555:errorcluster, "Device out"=w7554:refnum<class "Channel.lvclass">)  [unwired: 7 in]
            n3078 = call-dynamic "Write Channel.vi"("error in (no error)"=w7555, "Channel.lvclass"=w7554, "Acquisition in"=w7560) -> ("error out"=w7556:errorcluster, "Acquisition out"=w7558:refnum<class "Acquisition.lvclass">)  [unwired: 7 in]
            n3079 = call-dynamic "Write AcquisitionC.vi"("error in (no error)"=w7556, "Acquisition.lvclass"=w7558, "S4ACS_GUI in"=w7557) -> ("error out"=w7551:errorcluster, "S4ACS_GUI out"=w7550:refnum<class "S4GUI.lvclass">)  [unwired: 7 in]
          }
        }
      }
      event "Cooler 4": Value Change {
        n3080 = event-data() -> ("NewVal"=w7570:bool)  [unwired: 1 in]
        n3081 = case shown="True" w7570 {
          tunnel: w7574 -> [w7576 w7580]
          tunnel: w7573 -> [w7575 w7579]
          tunnel: [w7575 w7578] -> w7572
          tunnel: [w7576 w7577] -> w7571
          frame False {
          }
          frame True {
            n3082 = call-dynamic "Read AcquisitionD.vi"("error in (no error)"=w7579, "S4ACS_GUI in"=w7580) -> ("error out"=w7595:errorcluster, "Acquisition.lvclass"=w7596:refnum<class "Acquisition.lvclass">, "S4ACS_GUI out"=w7584:refnum<class "S4GUI.lvclass">)  [unwired: 7 in]
            n3083 = call-dynamic "Read Channel.vi"("error in (no error)"=w7595, "Acquisition in"=w7596) -> ("error out"=w7593:errorcluster, "Channel.lvclass"=w7594:refnum<class "Channel.lvclass">, "Acquisition out"=w7587:refnum<class "Acquisition.lvclass">)  [unwired: 7 in]
            n3084 = call-dynamic "Read State Machine.vi"("error in (no error)"=w7593, "Device in"=w7594) -> ("error out"=w7591:errorcluster, "State Machine.lvclass"=w7592:refnum<class "State Machine.lvclass">, "Device out"=w7588:refnum<class "Channel.lvclass">)  [unwired: 7 in]
            n3085 = call "Next State.vi"("error in (no error)"=w7591, "New_State"=u32 30, "State Machine in"=w7592) -> ("error out"=w7586:errorcluster, "State Machine out"=w7589:refnum<class "State Machine.lvclass">)  [unwired: 7 in]
            n3086 = call-dynamic "Write State Machine.vi"("error in (no error)"=w7586, "State Machine.lvclass"=w7589, "Device in"=w7588) -> ("error out"=w7582:errorcluster, "Device out"=w7581:refnum<class "Channel.lvclass">)  [unwired: 7 in]
            n3087 = call-dynamic "Write Channel.vi"("error in (no error)"=w7582, "Channel.lvclass"=w7581, "Acquisition in"=w7587) -> ("error out"=w7583:errorcluster, "Acquisition out"=w7585:refnum<class "Acquisition.lvclass">)  [unwired: 7 in]
            n3088 = call-dynamic "Write AcquisitionD.vi"("error in (no error)"=w7583, "Acquisition.lvclass"=w7585, "S4ACS_GUI in"=w7584) -> ("error out"=w7578:errorcluster, "S4ACS_GUI out"=w7577:refnum<class "S4GUI.lvclass">)  [unwired: 7 in]
          }
        }
      }
      event "Cooler status 4": Value Change {
        n3089 = event-data() -> ("NewVal"=w7597:bool)  [unwired: 1 in]
        n3090 = case shown="False" w7597 {
          tunnel: w7601 -> [w7610 w7623]
          tunnel: w7600 -> [w7609 w7622]
          tunnel: [w7608 w7622] -> w7599
          tunnel: [w7607 w7623] -> w7598
          frame False {
            n3091 = call-dynamic "Read AcquisitionD.vi"("error in (no error)"=w7609, "S4ACS_GUI in"=w7610) -> ("error out"=w7620:errorcluster, "Acquisition.lvclass"=w7621:refnum<class "Acquisition.lvclass">, "S4ACS_GUI out"=w7614:refnum<class "S4GUI.lvclass">)  [unwired: 7 in]
            n3092 = call-dynamic "Read Channel.vi"("error in (no error)"=w7620, "Acquisition in"=w7621) -> ("error out"=w7618:errorcluster, "Channel.lvclass"=w7619:refnum<class "Channel.lvclass">, "Acquisition out"=w7616:refnum<class "Acquisition.lvclass">)  [unwired: 7 in]
            n3093 = call-dynamic "Read State Machine.vi"("error in (no error)"=w7618, "Device in"=w7619) -> ("error out"=w7604:errorcluster, "State Machine.lvclass"=w7606:refnum<class "State Machine.lvclass">, "Device out"=w7617:refnum<class "Channel.lvclass">)  [unwired: 7 in]
            n3094 = call-dynamic "Read Previous State.vi"("error in (no error)"=w7604, "State Machine in"=w7606) -> ("error out"=w7603:errorcluster, "Previous State"=→"State":dbl, "State Machine out"=w7605:refnum<class "State Machine.lvclass">)  [unwired: 7 in]
            n3095 = call-dynamic "Write State Machine.vi"("error in (no error)"=w7603, "State Machine.lvclass"=w7605, "Device in"=w7617) -> ("error out"=w7612:errorcluster, "Device out"=w7611:refnum<class "Channel.lvclass">)  [unwired: 7 in]
            n3096 = call-dynamic "Write Channel.vi"("error in (no error)"=w7612, "Channel.lvclass"=w7611, "Acquisition in"=w7616) -> ("error out"=w7613:errorcluster, "Acquisition out"=w7615:refnum<class "Acquisition.lvclass">)  [unwired: 7 in]
            n3097 = call-dynamic "Write AcquisitionD.vi"("error in (no error)"=w7613, "Acquisition.lvclass"=w7615, "S4ACS_GUI in"=w7614) -> ("error out"=w7608:errorcluster, "S4ACS_GUI out"=w7607:refnum<class "S4GUI.lvclass">)  [unwired: 7 in]
          }
          frame True {
          }
        }
      }
      event "Set Temp 1": Value Change {
        n3098 = event-data() -> ("NewVal"=w7624:bool)  [unwired: 1 in]
        n3099 = case shown="True" w7624 {
          tunnel: w7628 -> [w7630 w7644]
          tunnel: w7627 -> [w7629 w7643]
          tunnel: [w7629 w7642] -> w7626
          tunnel: [w7630 w7641] -> w7625
          frame False {
          }
          frame True {
            n3100 = call-dynamic "Read AcquisitionA.vi"("error in (no error)"=w7643, "S4ACS_GUI in"=w7644) -> ("error out"=w7657:errorcluster, "Acquisition.lvclass"=w7658:refnum<class "Acquisition.lvclass">, "S4ACS_GUI out"=w7648:refnum<class "S4GUI.lvclass">)  [unwired: 7 in]
            n3101 = call-dynamic "Read Channel.vi"("error in (no error)"=w7657, "Acquisition in"=w7658) -> ("error out"=w7639:errorcluster, "Channel.lvclass"=w7640:refnum<class "Channel.lvclass">, "Acquisition out"=w7651:refnum<class "Acquisition.lvclass">)  [unwired: 7 in]
            n3102 = call-dynamic "Read Interface.vi"("error in (no error)"=w7639, "Channel in"=w7640) -> ("error out"=w7637:errorcluster, "Interface.lvclass"=w7638:refnum<class "Interface.lvclass">, "Channel out"=w7635:refnum<class "Channel.lvclass">)  [unwired: 7 in]
            n3103 = call-dynamic "Write Temperature.vi"("error in (no error)"=w7637, "Temperature"="Target Temp 1", "Interface in"=w7638) -> ("error out"=w7633:errorcluster, "Interface out"=w7636:refnum<class "Interface.lvclass">)  [unwired: 7 in]
            n3104 = call-dynamic "Write Interface.vi"("error in (no error)"=w7633, "Interface.lvclass"=w7636, "Channel in"=w7635) -> ("error out"=w7632:errorcluster, "Channel out"=w7634:refnum<class "Channel.lvclass">)  [unwired: 7 in]
            n3105 = call-dynamic "Read State Machine.vi"("error in (no error)"=w7632, "Device in"=w7634) -> ("error out"=w7655:errorcluster, "State Machine.lvclass"=w7656:refnum<class "State Machine.lvclass">, "Device out"=w7652:refnum<class "Channel.lvclass">)  [unwired: 7 in]
            n3106 = call "Next State.vi"("error in (no error)"=w7655, "New_State"=u32 35, "State Machine in"=w7656) -> ("error out"=w7650:errorcluster, "State Machine out"=w7653:refnum<class "State Machine.lvclass">)  [unwired: 7 in]
            n3107 = call-dynamic "Write State Machine.vi"("error in (no error)"=w7650, "State Machine.lvclass"=w7653, "Device in"=w7652) -> ("error out"=w7646:errorcluster, "Device out"=w7645:refnum<class "Channel.lvclass">)  [unwired: 7 in]
            n3108 = call-dynamic "Write Channel.vi"("error in (no error)"=w7646, "Channel.lvclass"=w7645, "Acquisition in"=w7651) -> ("error out"=w7647:errorcluster, "Acquisition out"=w7649:refnum<class "Acquisition.lvclass">)  [unwired: 7 in]
            n3109 = call-dynamic "Write AcquisitionA.vi"("error in (no error)"=w7647, "Acquisition.lvclass"=w7649, "S4ACS_GUI in"=w7648) -> ("error out"=w7642:errorcluster, "S4ACS_GUI out"=w7641:refnum<class "S4GUI.lvclass">)  [unwired: 7 in]
          }
        }
      }
      event "Set Temp 2": Value Change {
        n3110 = event-data() -> ("NewVal"=w7659:bool)  [unwired: 1 in]
        n3111 = case shown="True" w7659 {
          tunnel: w7663 -> [w7665 w7679]
          tunnel: w7662 -> [w7664 w7678]
          tunnel: [w7664 w7677] -> w7661
          tunnel: [w7665 w7676] -> w7660
          frame False {
          }
          frame True {
            n3112 = call "Read AcquisitionB.vi"("error in (no error)"=w7678, "S4ACS_GUI in"=w7679) -> ("error out"=w7692:errorcluster, "Acquisition.lvclass"=w7693:refnum<class "Acquisition.lvclass">, "S4ACS_GUI out"=w7683:refnum<class "S4GUI.lvclass">)  [unwired: 7 in]
            n3113 = call-dynamic "Read Channel.vi"("error in (no error)"=w7692, "Acquisition in"=w7693) -> ("error out"=w7674:errorcluster, "Channel.lvclass"=w7675:refnum<class "Channel.lvclass">, "Acquisition out"=w7686:refnum<class "Acquisition.lvclass">)  [unwired: 7 in]
            n3114 = call-dynamic "Read Interface.vi"("error in (no error)"=w7674, "Channel in"=w7675) -> ("error out"=w7672:errorcluster, "Interface.lvclass"=w7673:refnum<class "Interface.lvclass">, "Channel out"=w7670:refnum<class "Channel.lvclass">)  [unwired: 7 in]
            n3115 = call-dynamic "Write Temperature.vi"("error in (no error)"=w7672, "Temperature"="Target Temp 2", "Interface in"=w7673) -> ("error out"=w7668:errorcluster, "Interface out"=w7671:refnum<class "Interface.lvclass">)  [unwired: 7 in]
            n3116 = call-dynamic "Write Interface.vi"("error in (no error)"=w7668, "Interface.lvclass"=w7671, "Channel in"=w7670) -> ("error out"=w7667:errorcluster, "Channel out"=w7669:refnum<class "Channel.lvclass">)  [unwired: 7 in]
            n3117 = call-dynamic "Read State Machine.vi"("error in (no error)"=w7667, "Device in"=w7669) -> ("error out"=w7690:errorcluster, "State Machine.lvclass"=w7691:refnum<class "State Machine.lvclass">, "Device out"=w7687:refnum<class "Channel.lvclass">)  [unwired: 7 in]
            n3118 = call "Next State.vi"("error in (no error)"=w7690, "New_State"=u32 35, "State Machine in"=w7691) -> ("error out"=w7685:errorcluster, "State Machine out"=w7688:refnum<class "State Machine.lvclass">)  [unwired: 7 in]
            n3119 = call-dynamic "Write State Machine.vi"("error in (no error)"=w7685, "State Machine.lvclass"=w7688, "Device in"=w7687) -> ("error out"=w7681:errorcluster, "Device out"=w7680:refnum<class "Channel.lvclass">)  [unwired: 7 in]
            n3120 = call-dynamic "Write Channel.vi"("error in (no error)"=w7681, "Channel.lvclass"=w7680, "Acquisition in"=w7686) -> ("error out"=w7682:errorcluster, "Acquisition out"=w7684:refnum<class "Acquisition.lvclass">)  [unwired: 7 in]
            n3121 = call "Write AcquisitionB.vi"("error in (no error)"=w7682, "Acquisition.lvclass"=w7684, "S4ACS_GUI in"=w7683) -> ("error out"=w7677:errorcluster, "S4ACS_GUI out"=w7676:refnum<class "S4GUI.lvclass">)  [unwired: 7 in]
          }
        }
      }
      event "Set Temp 3": Value Change {
        n3122 = event-data() -> ("NewVal"=w7694:bool)  [unwired: 1 in]
        n3123 = case shown="True" w7694 {
          tunnel: w7698 -> [w7700 w7714]
          tunnel: w7697 -> [w7699 w7713]
          tunnel: [w7699 w7712] -> w7696
          tunnel: [w7700 w7711] -> w7695
          frame False {
          }
          frame True {
            n3124 = call-dynamic "Read AcquisitionC.vi"("error in (no error)"=w7713, "S4ACS_GUI in"=w7714) -> ("error out"=w7727:errorcluster, "Acquisition.lvclass"=w7728:refnum<class "Acquisition.lvclass">, "S4ACS_GUI out"=w7718:refnum<class "S4GUI.lvclass">)  [unwired: 7 in]
            n3125 = call-dynamic "Read Channel.vi"("error in (no error)"=w7727, "Acquisition in"=w7728) -> ("error out"=w7709:errorcluster, "Channel.lvclass"=w7710:refnum<class "Channel.lvclass">, "Acquisition out"=w7721:refnum<class "Acquisition.lvclass">)  [unwired: 7 in]
            n3126 = call-dynamic "Read Interface.vi"("error in (no error)"=w7709, "Channel in"=w7710) -> ("error out"=w7707:errorcluster, "Interface.lvclass"=w7708:refnum<class "Interface.lvclass">, "Channel out"=w7705:refnum<class "Channel.lvclass">)  [unwired: 7 in]
            n3127 = call-dynamic "Write Temperature.vi"("error in (no error)"=w7707, "Temperature"="Target Temp 3", "Interface in"=w7708) -> ("error out"=w7703:errorcluster, "Interface out"=w7706:refnum<class "Interface.lvclass">)  [unwired: 7 in]
            n3128 = call-dynamic "Write Interface.vi"("error in (no error)"=w7703, "Interface.lvclass"=w7706, "Channel in"=w7705) -> ("error out"=w7702:errorcluster, "Channel out"=w7704:refnum<class "Channel.lvclass">)  [unwired: 7 in]
